vi "AOTF_frequency _Initialization3.vi"() -> ()   [LabVIEW 2009]
uses:
  <userlib>/AotfLibrary/AotfLibrary.lvlib
panel:
  out "concatenated string 2":string
  out "concatenated string":string
  out "concatenated string 7":string
  out "concatenated string 6":string
  out "concatenated string 5":string
  out "concatenated string 4":string
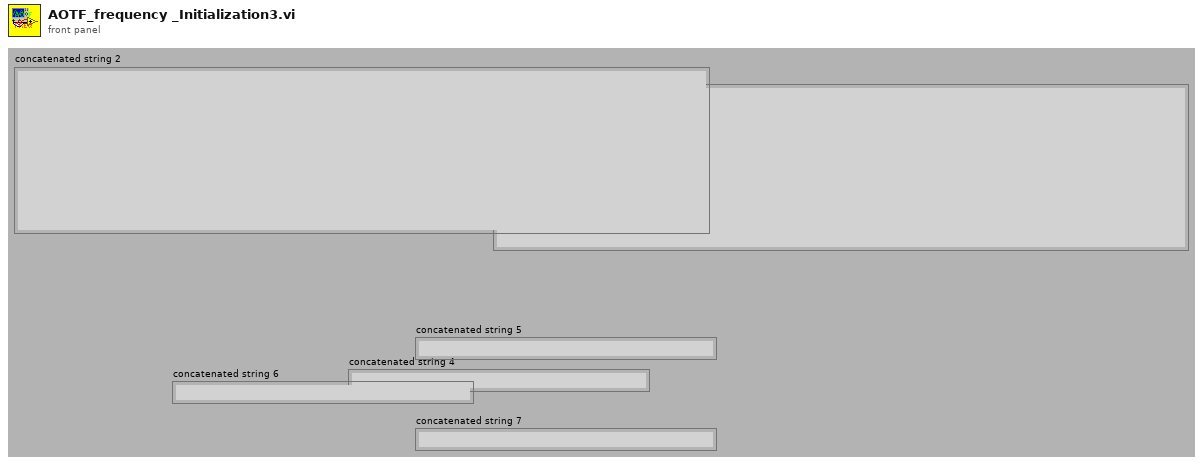
[diagram p1: front panel]
types:
  T1 = typedef "AOTFSettings.ctt" = cluster{"Laser 1 Output Channel":tag, "AOTF  1 Output Voltage":dbl, "Laser 2 Output Channel":tag, "AOTF  2 Output Voltage":dbl, "Laser 3 Output Channel":tag, "AOTF  3 Output Voltage":dbl, "Pixel per Cycle":u16, "Time per Cycle  / ms":dbl, "Laser 4 Output Channel":tag, "AOTF  4 Output Voltage":dbl, "Laser 5 Output Channel":tag, "AOTF 5 Output Voltage ":dbl, "Laser 6 Output Channel":tag, "AOTF  6 Output Voltage ":dbl, "Laser 7 Output Channel":tag, "AOTF 7 Output Voltage ":dbl, "Laser 8 Output Channel":tag, "AOTF  8 Output Voltage ":dbl, "AOTF  1 Frequency":dbl, "AOTF  2 Frequency":dbl, "AOTF  3  Frequency":dbl, "AOTF  4 Frequency":dbl, "AOTF 5 Frequency":dbl, "AOTF  6 Frequency":dbl, "AOTF 7  Frequency":dbl, "AOTF  8 Frequency":dbl, "AOTF  1 Amplitude":dbl, "AOTF  2 Amplitude":dbl, "AOTF  3  Amplitude":dbl, "AOTF  4 Amplitude":dbl, "AOTF 5 Amplitude":dbl, "AOTF  6 Amplitude":dbl, "AOTF 7 Amplitude  ":dbl, "AOTF  8 Amplitude":dbl}
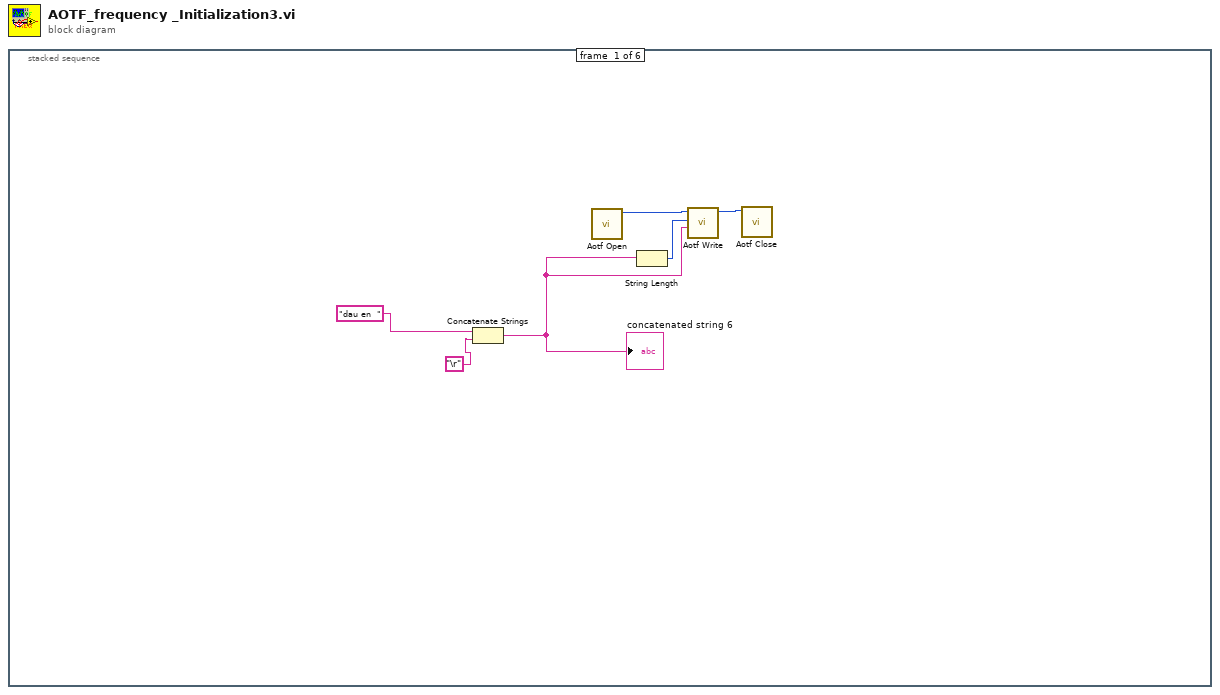
[diagram p0: block diagram]
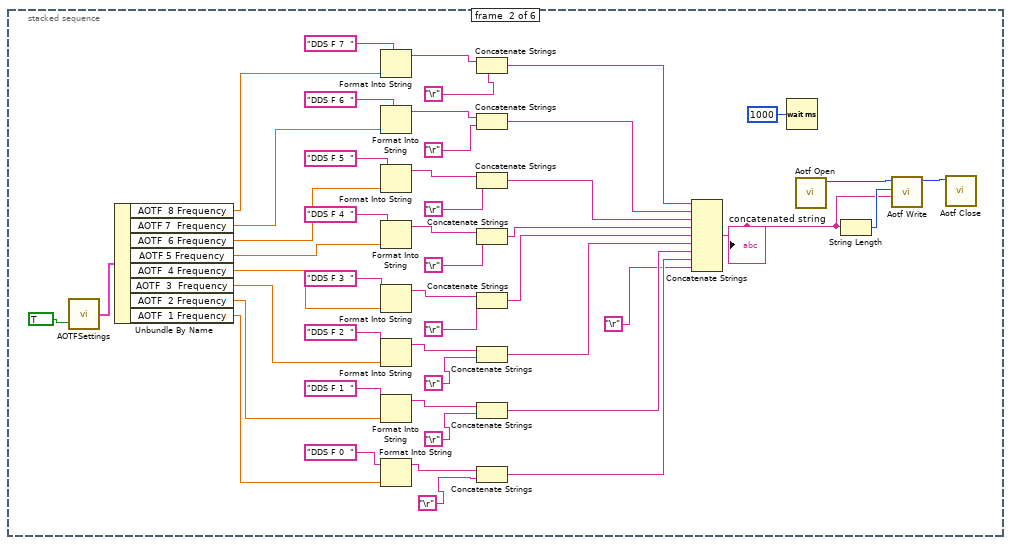
[diagram p2: hidden frame]
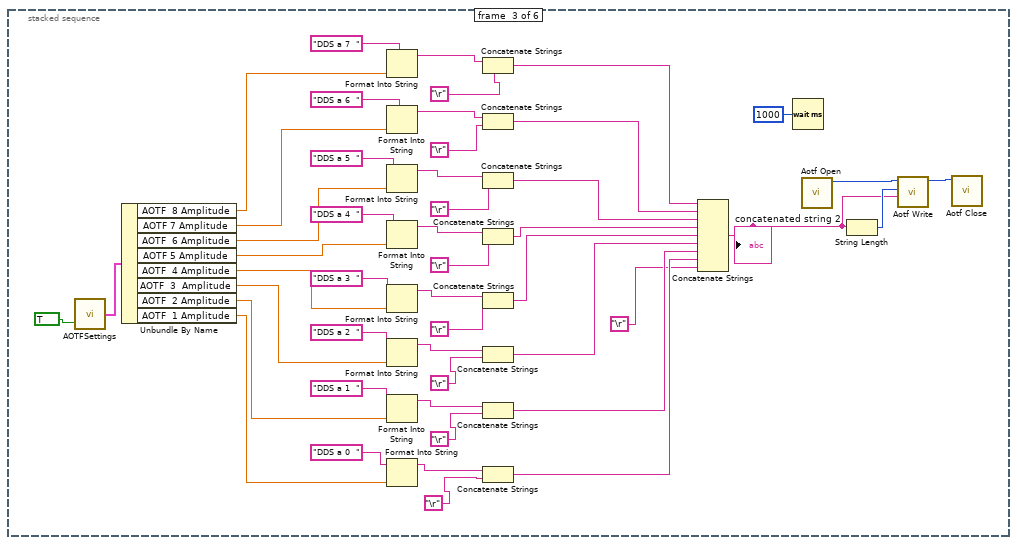
[diagram p3: hidden frame]
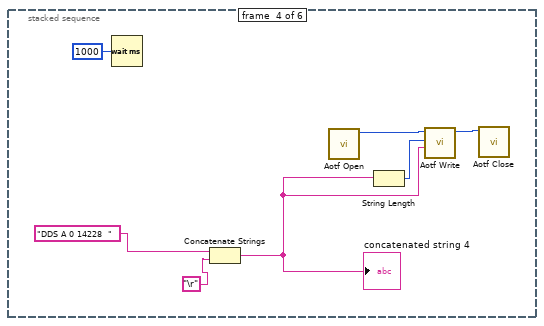
[diagram p4: hidden frame]
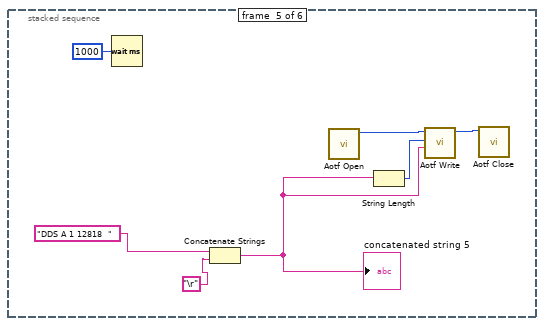
[diagram p5: hidden frame]
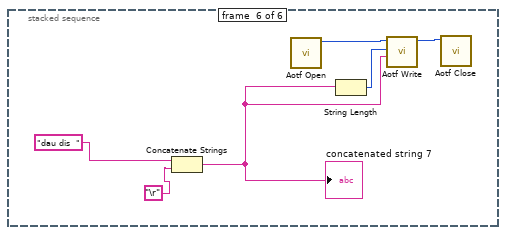
[diagram p6: hidden frame]
diagram:
  n1 = stacked-sequence {
    frame #0 {
      n2 = Concatenate Strings("dau en  " ("string"), "\r") -> (w2:string)
      "concatenated string 6" <- w2
      n3 = call <userlib>:"Aotf Open.vi"() -> ("function return"=w5:u32)  [unwired: 11 in]
      n4 = String Length(string=w2) -> (length=w4:i32)
      n5 = call <userlib>:"Aotf Write.vi"("pData"=w2, "uiLength"=w4, "hAotfController"=w5) -> ("hAotfController out"=w6:u32)  [unwired: 7 in, 1 out]
      n6 = call <userlib>:"Aotf Close.vi"("hAotfController"=w6) -> ()  [unwired: 9 in, 2 out]
    }
    frame #1 {
      n7 = call "AOTFSettings.vi"("Get/Set"=TRUE) -> ("AOTF Setting (Output)"=w52:T1)  [unwired: 1 in]
      n8 = Unbundle By Name(w52) -> ("AOTF  8 Frequency"=w28:dbl, "AOTF 7  Frequency"=w27:dbl, "AOTF  6 Frequency"=w26:dbl, "AOTF 5 Frequency"=w25:dbl, "AOTF  4 Frequency"=w21:dbl, "AOTF  3  Frequency"=w22:dbl, "AOTF  2 Frequency"=w23:dbl, "AOTF  1 Frequency"=w24:dbl)
      n9 = Format Into String(initial string="DDS F 7  " ("string"), w28) -> (resulting string=w31:string)  [unwired: 2 in, 1 out]
      n10 = Format Into String(initial string="DDS F 6  " ("string"), w27) -> (resulting string=w33:string)  [unwired: 2 in, 1 out]
      n11 = Format Into String(initial string="DDS F 5  " ("string"), w26) -> (resulting string=w36:string)  [unwired: 2 in, 1 out]
      n12 = Format Into String(initial string="DDS F 4  " ("string"), w25) -> (resulting string=w39:string)  [unwired: 2 in, 1 out]
      n13 = Format Into String(initial string="DDS F 3  " ("string"), w21) -> (resulting string=w42:string)  [unwired: 2 in, 1 out]
      n14 = Format Into String(initial string="DDS F 2  " ("string"), w22) -> (resulting string=w45:string)  [unwired: 2 in, 1 out]
      n15 = Format Into String(initial string="DDS F 1  " ("string"), w23) -> (resulting string=w48:string)  [unwired: 2 in, 1 out]
      n16 = Format Into String(initial string="DDS F 0  " ("string"), w24) -> (resulting string=w54:string)  [unwired: 2 in, 1 out]
      n17 = Concatenate Strings(w31, "\r") -> (w16:string)
      n18 = Concatenate Strings(w33, "\r") -> (w17:string)
      n19 = Concatenate Strings(w36, "\r") -> (w18:string)
      n20 = Concatenate Strings(w39, "\r") -> (w19:string)
      n21 = Concatenate Strings(w42, "\r") -> (w15:string)
      n22 = Concatenate Strings(w45, "\r") -> (w13:string)
      n23 = Concatenate Strings(w48, "\r") -> (w12:string)
      n24 = Concatenate Strings(w54, "\r") -> (w14:string)
      n25 = Concatenate Strings(w16, w17, w18, w19, w15, w13, w12, w14, "\r") -> (w7:string)
      "concatenated string" <- w7
      n26 = Wait (ms)(milliseconds to wait=u32 1000) -> ()  [unwired: 1 out]
      n27 = call <userlib>:"Aotf Open.vi"() -> ("function return"=w9:u32)  [unwired: 11 in]
      n28 = String Length(string=w7) -> (length=w10:i32)
      n29 = call <userlib>:"Aotf Write.vi"("pData"=w7, "uiLength"=w10, "hAotfController"=w9) -> ("hAotfController out"=w8:u32)  [unwired: 7 in, 1 out]
      n30 = call <userlib>:"Aotf Close.vi"("hAotfController"=w8) -> ()  [unwired: 9 in, 2 out]
    }
    frame #2 {
      n31 = call "AOTFSettings.vi"("Get/Set"=TRUE) -> ("AOTF Setting (Output)"=w100:T1)  [unwired: 1 in]
      n32 = Unbundle By Name(w100) -> ("AOTF  8 Amplitude"=w76:dbl, "AOTF 7 Amplitude"=w75:dbl, "AOTF  6 Amplitude"=w74:dbl, "AOTF 5 Amplitude"=w73:dbl, "AOTF  4 Amplitude"=w69:dbl, "AOTF  3  Amplitude"=w70:dbl, "AOTF  2 Amplitude"=w71:dbl, "AOTF  1 Amplitude"=w72:dbl)
      n33 = Format Into String(initial string="DDS a 7  " ("string"), w76) -> (resulting string=w79:string)  [unwired: 2 in, 1 out]
      n34 = Format Into String(initial string="DDS a 6  " ("string"), w75) -> (resulting string=w81:string)  [unwired: 2 in, 1 out]
      n35 = Format Into String(initial string="DDS a 5  " ("string"), w74) -> (resulting string=w84:string)  [unwired: 2 in, 1 out]
      n36 = Format Into String(initial string="DDS a 4  " ("string"), w73) -> (resulting string=w87:string)  [unwired: 2 in, 1 out]
      n37 = Format Into String(initial string="DDS a 3  " ("string"), w69) -> (resulting string=w90:string)  [unwired: 2 in, 1 out]
      n38 = Format Into String(initial string="DDS a 2  " ("string"), w70) -> (resulting string=w93:string)  [unwired: 2 in, 1 out]
      n39 = Format Into String(initial string="DDS a 1  " ("string"), w71) -> (resulting string=w96:string)  [unwired: 2 in, 1 out]
      n40 = Format Into String(initial string="DDS a 0  " ("string"), w72) -> (resulting string=w102:string)  [unwired: 2 in, 1 out]
      n41 = Concatenate Strings(w79, "\r") -> (w64:string)
      n42 = Concatenate Strings(w81, "\r") -> (w65:string)
      n43 = Concatenate Strings(w84, "\r") -> (w66:string)
      n44 = Concatenate Strings(w87, "\r") -> (w67:string)
      n45 = Concatenate Strings(w90, "\r") -> (w63:string)
      n46 = Concatenate Strings(w93, "\r") -> (w61:string)
      n47 = Concatenate Strings(w96, "\r") -> (w60:string)
      n48 = Concatenate Strings(w102, "\r") -> (w62:string)
      n49 = Concatenate Strings(w64, w65, w66, w67, w63, w61, w60, w62, "\r") -> (w55:string)
      "concatenated string 2" <- w55
      n50 = Wait (ms)(milliseconds to wait=u32 1000) -> ()  [unwired: 1 out]
      n51 = call <userlib>:"Aotf Open.vi"() -> ("function return"=w57:u32)  [unwired: 11 in]
      n52 = String Length(string=w55) -> (length=w58:i32)
      n53 = call <userlib>:"Aotf Write.vi"("pData"=w55, "uiLength"=w58, "hAotfController"=w57) -> ("hAotfController out"=w56:u32)  [unwired: 7 in, 1 out]
      n54 = call <userlib>:"Aotf Close.vi"("hAotfController"=w56) -> ()  [unwired: 9 in, 2 out]
    }
    frame #3 {
      n55 = Wait (ms)(milliseconds to wait=u32 1000) -> ()  [unwired: 1 out]
      n56 = Concatenate Strings("DDS A 0 14228  " ("string"), "\r") -> (w105:string)
      "concatenated string 4" <- w105
      n57 = call <userlib>:"Aotf Open.vi"() -> ("function return"=w108:u32)  [unwired: 11 in]
      n58 = String Length(string=w105) -> (length=w107:i32)
      n59 = call <userlib>:"Aotf Write.vi"("pData"=w105, "uiLength"=w107, "hAotfController"=w108) -> ("hAotfController out"=w109:u32)  [unwired: 7 in, 1 out]
      n60 = call <userlib>:"Aotf Close.vi"("hAotfController"=w109) -> ()  [unwired: 9 in, 2 out]
    }
    frame #4 {
      n61 = Wait (ms)(milliseconds to wait=u32 1000) -> ()  [unwired: 1 out]
      n62 = Concatenate Strings("DDS A 1 12818  " ("string"), "\r") -> (w112:string)
      "concatenated string 5" <- w112
      n63 = call <userlib>:"Aotf Open.vi"() -> ("function return"=w115:u32)  [unwired: 11 in]
      n64 = String Length(string=w112) -> (length=w114:i32)
      n65 = call <userlib>:"Aotf Write.vi"("pData"=w112, "uiLength"=w114, "hAotfController"=w115) -> ("hAotfController out"=w116:u32)  [unwired: 7 in, 1 out]
      n66 = call <userlib>:"Aotf Close.vi"("hAotfController"=w116) -> ()  [unwired: 9 in, 2 out]
    }
    frame #5 {
      n67 = Concatenate Strings("dau dis  " ("string"), "\r") -> (w118:string)
      "concatenated string 7" <- w118
      n68 = call <userlib>:"Aotf Open.vi"() -> ("function return"=w121:u32)  [unwired: 11 in]
      n69 = String Length(string=w118) -> (length=w120:i32)
      n70 = call <userlib>:"Aotf Write.vi"("pData"=w118, "uiLength"=w120, "hAotfController"=w121) -> ("hAotfController out"=w122:u32)  [unwired: 7 in, 1 out]
      n71 = call <userlib>:"Aotf Close.vi"("hAotfController"=w122) -> ()  [unwired: 9 in, 2 out]
    }
  }
